vi "Generacion.vi"() -> ()   [LabVIEW 2016]
uses:
  <vilib>/sound2/lvsound2.llb/Sound Data Format.ctl
  <vilib>/sound2/lvsound2.llb/Sampling Mode.ctl
  <vilib>/measure/NI_MABase.lvlib
  <vilib>/Waveform/WDTOps.llb/WDT Append Waveforms DBL.vi
  <vilib>/sound2/lvsound2.llb/Sound File Write (DBL Single).vi
  <vilib>/sound2/lvsound2.llb/Sound File Write Open.vi
  <vilib>/sound2/lvsound2.llb/Sound Output Write (DBL Single).vi
panel:
  out "size(s)":i32
  in  "Normalizar":bool caption="Normalizar amplitud"
  in  "Tipo fichero":T1(ring)
  in  "Generar":bool
  in  "Reproducir":bool
  in  "Exit":bool
  in  "Salvar":bool
  in  "Ruido":bool
  in  "A_ruido":dbl=0.1 caption="Amplitud ruido"
  in  "Tipo_portadora":T2(ring) caption="Tipo portadora"
  in  "A_portadora":dbl=0.7 caption="Amplitud portadora" min=0.0 max=1.0
  in  "T_portadoras":dbl[](array[numeric])=[100.0, 150.0, 100.0, 150.0, 100.0, 150.0, 100.0] caption="Tiempo entre portadoras (ms)"
  out "Señal":waveform(dbl)(graph)
  in  "Duración":dbl=5.0 caption="Duración portadora (ms)"
  in  "Muestreo":dbl=48000.0 caption="Muestreo (muestras/s)"
  in  "F_portadora":dbl=1000.0 caption="Frecuencia portadora (Hz)" format="%#_13g"
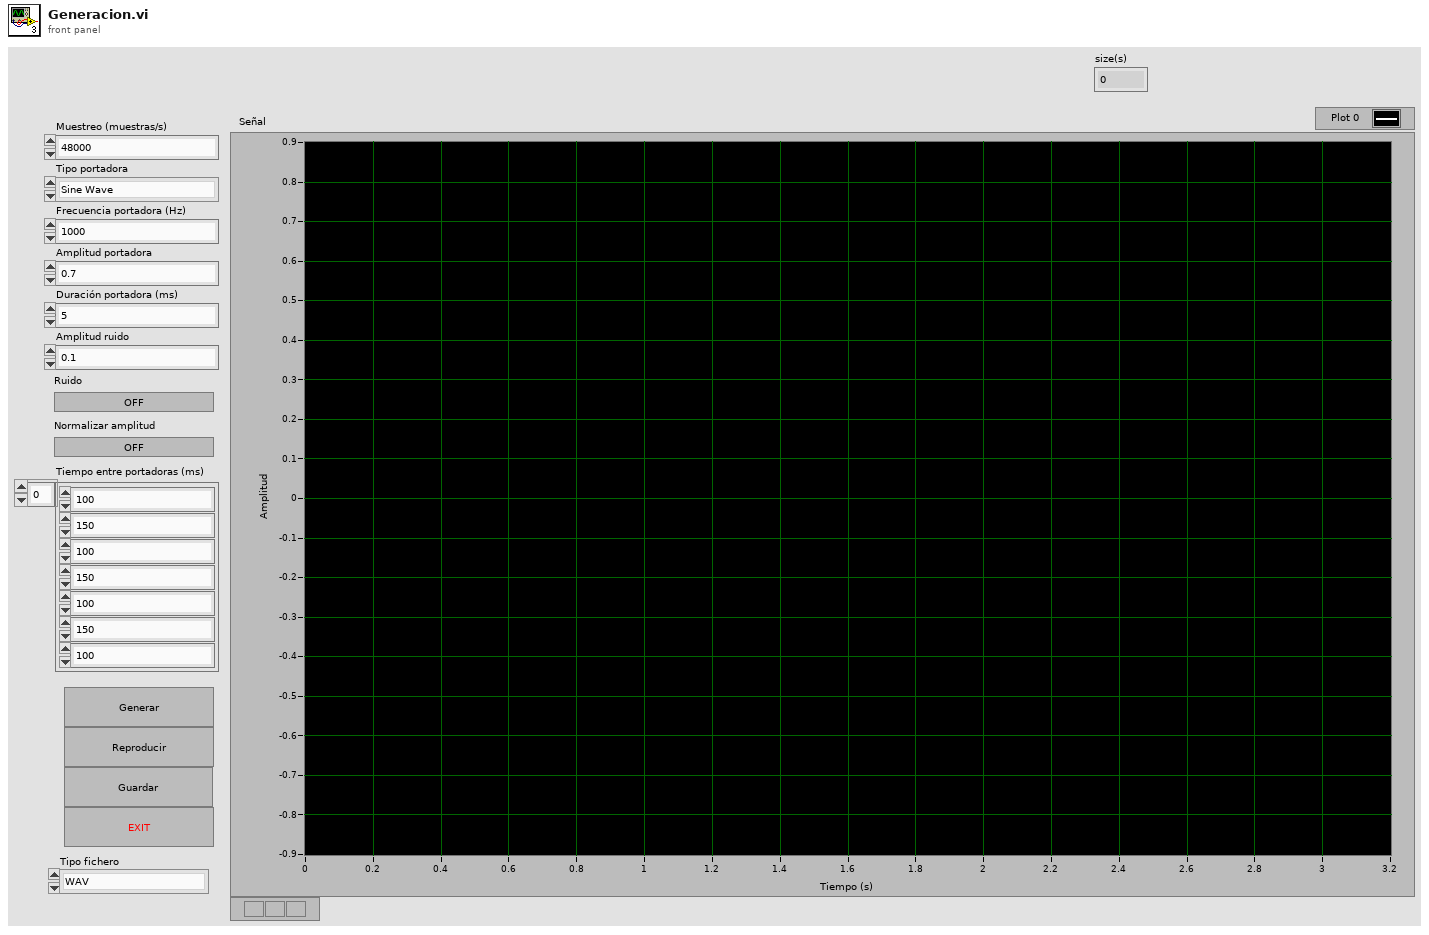
[diagram p1: front panel]
types:
  T1 = enum16{"WAV", "Bin 16 bits, little-endian", "Bin 16 bits, big-endian"}
  T2 = enum16{"Sine Wave", "Triangle Wave", "Square Wave", "Sawtooth Wave"}
  T3 = typedef "Sound Data Format.ctl" = cluster{"sample rate (S/s)":dbl, "number of channels":i32, "bits per sample":i32}
  T4 = enum16{"big-endian, network order", "native, host order", "little-endian"}
  T5 = enum16{"open", "replace", "create", "open or create", "replace or create", "replace or create with confirmation"}
  T6 = typedef "Sound File Refnum.ctl" = refnum<file>
  T7 = typedef "Sampling Mode.ctl" = i32
  T8 = typedef "Sound Output Task ID.ctl" = u32
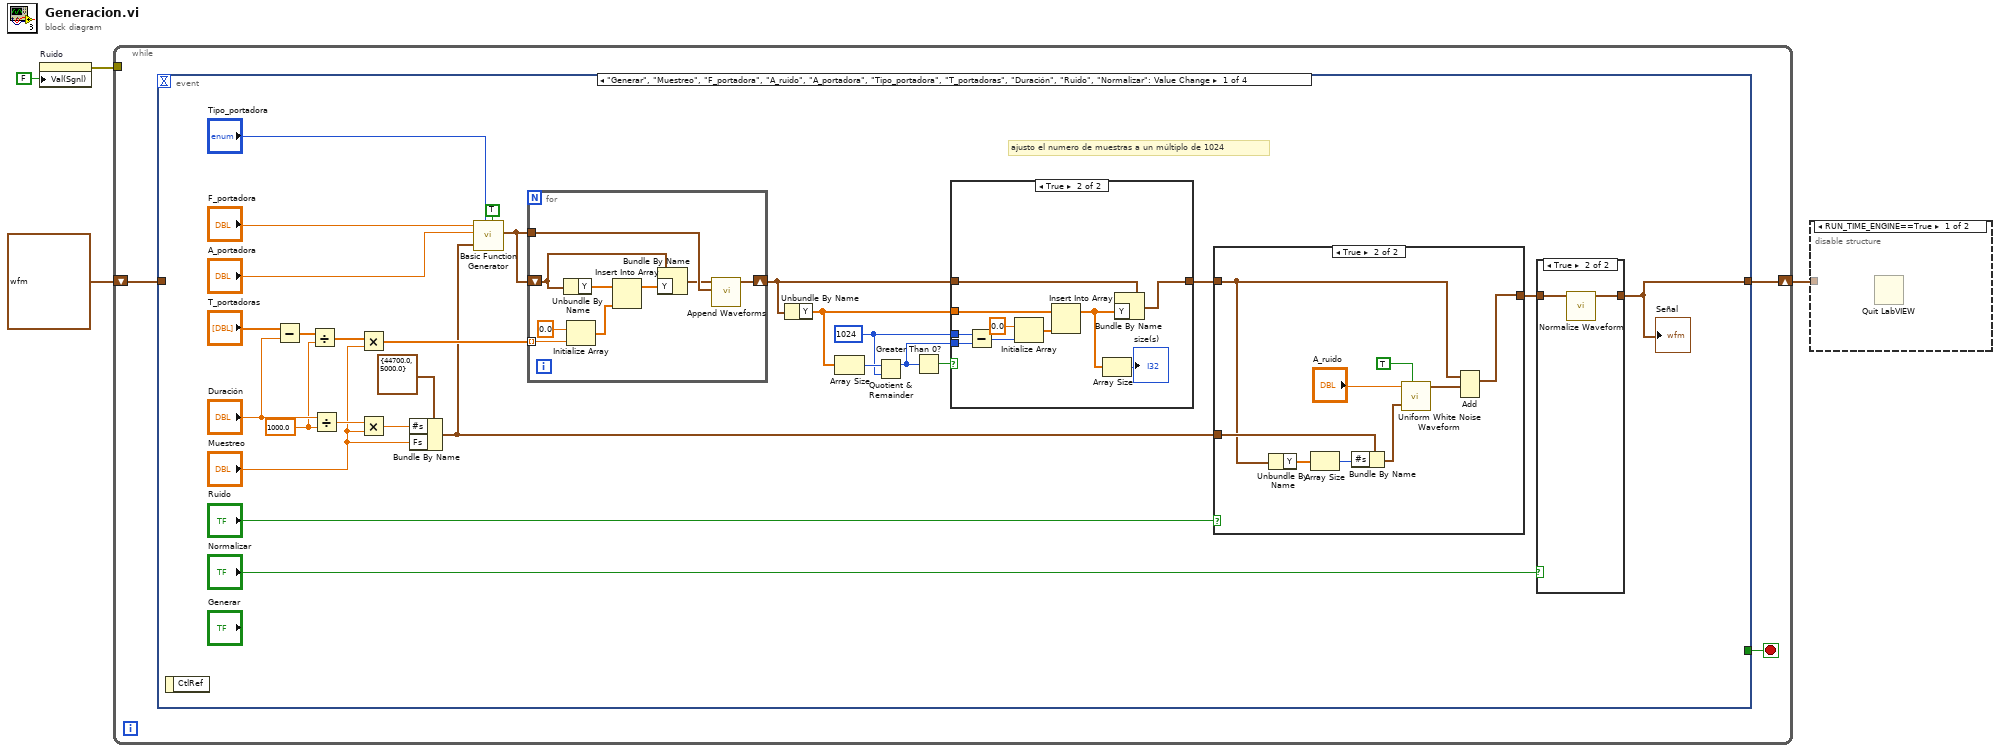
[diagram p0: block diagram]
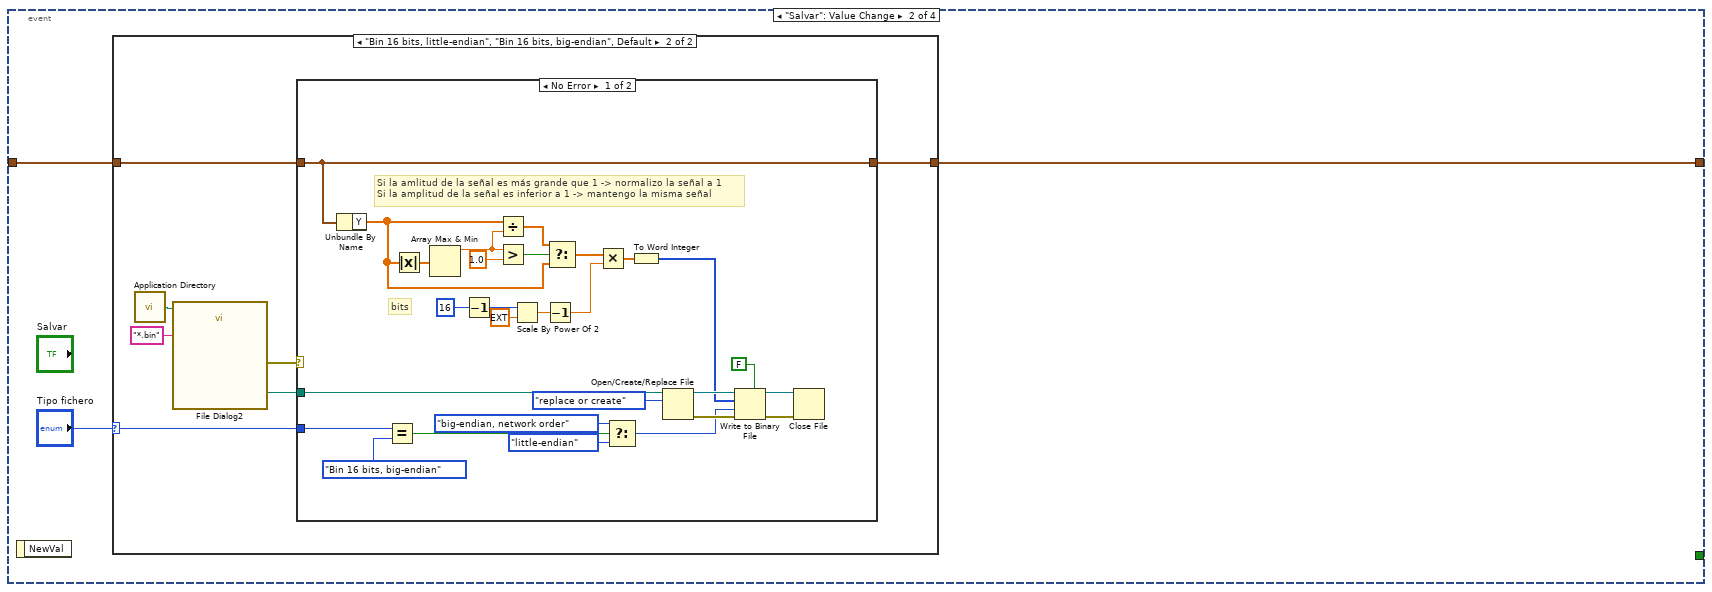
[diagram p6: hidden frame]
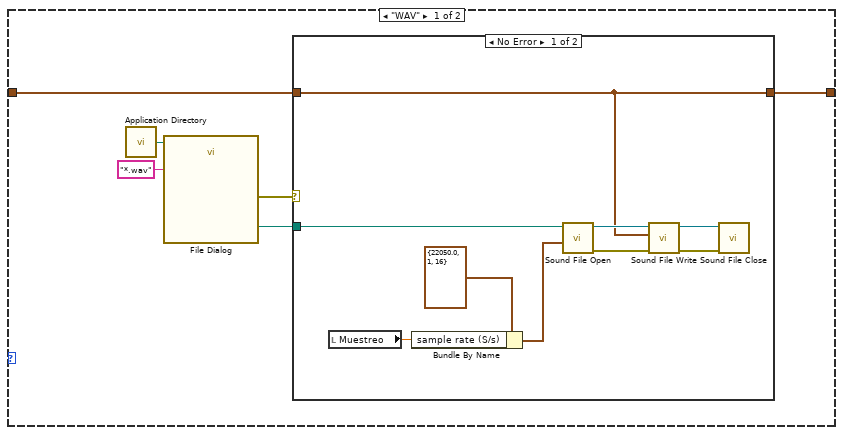
[diagram p7: hidden frame]
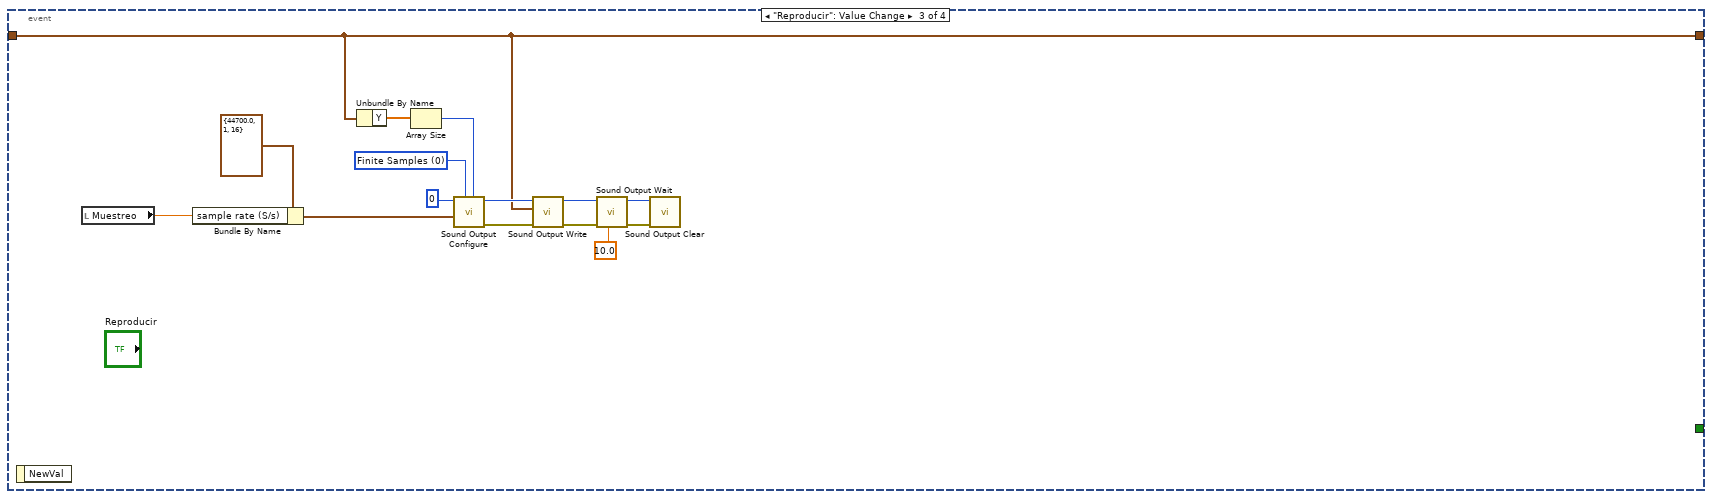
[diagram p10: hidden frame]
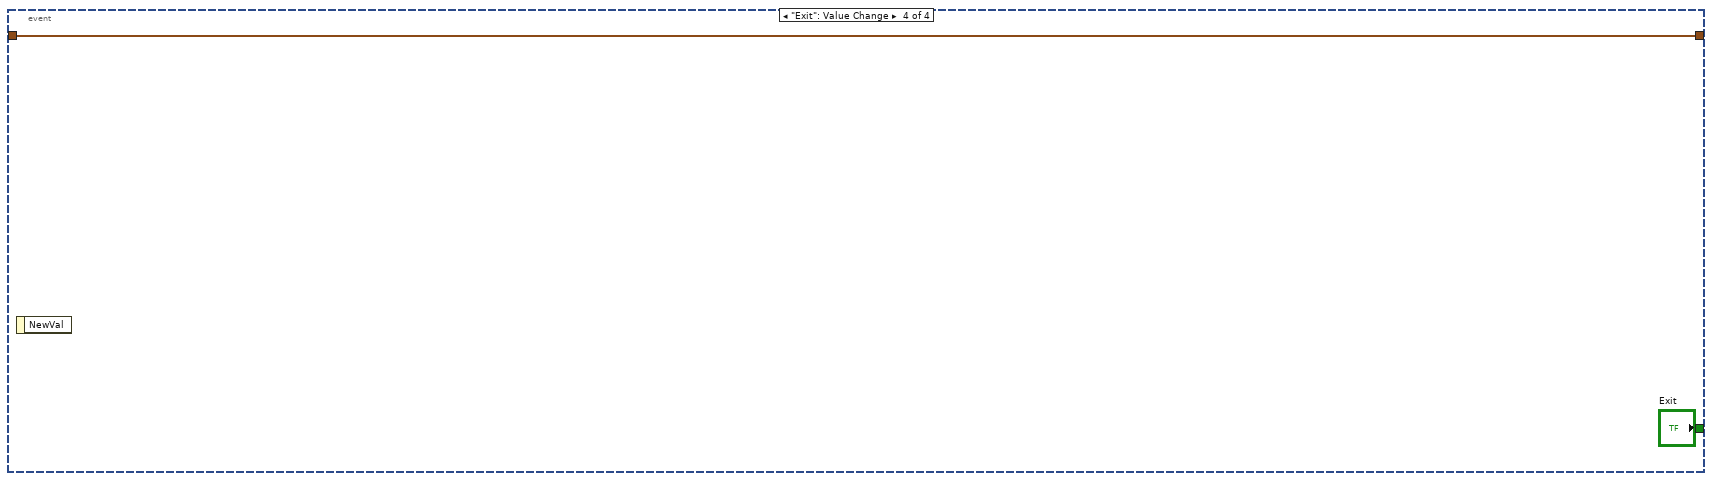
[diagram p11: hidden frame]
diagram:
  n1 = property on="Ruido" class="Bool (strict)"("Val(Sgnl)"=FALSE ("Value (Signaling)")) -> (error out=w3:errorcluster)  [unwired: 2 in, 1 out]
  n2 = while {
    shift-right: [w6] -> w1
    shift-left: waveform(dbl) {"t0"=timestamp(0 s since 1904-01-01), "dt"=1.0, "Y"=[]} ("signal out") -> [w5]
    tunnel: w3 -> [_]
    stop <- w7 stop-if-true
    n3 = event shown="[0] \"Generar\", \"Muestreo\", \"F_portadora\", \"A_ruido\", \"A_portadora\", \"Tipo_portadora\", \"T_portadoras\", \"Duración\", \"Ruido\", \"Normalizar\": Value Change" {
      selector: _ -> [_ _ _ _]
      dyn-events: _ -> [_ _ _ _]
      timeout: _ -> [_ _ _ _]
      tunnel: [_ _ _ "Exit"] -> w7
      tunnel: [w17 w68 w126 w138] -> w6
      tunnel: w5 -> [_ w69 w126 w138]
      event "Generar", "Muestreo", "F_portadora", "A_ruido", "A_portadora", "Tipo_portadora", "T_portadoras", "Duración", "Ruido", "Normalizar": Value Change {
        w8 = 1024 ("y")
        w16 = 1000.0 ("y")
        # "ajusto el numero de muestras a un múltiplo de 1024"
        n4 = event-data() -> ()  [unwired: 1 in, 1 out]
        n5 = Subtract(x="T_portadoras", y="Duración") -> (x-y=w28:dbl[])
        n6 = Divide(x=w28, y=w16) -> (x/y=w32:dbl[])
        n7 = Divide(x="Duración", y=w16) -> (x/y=w34:dbl)
        n8 = Multiply(x=w32, y="Muestreo") -> (x*y=w31:dbl[])
        n9 = Multiply(x=w34, y="Muestreo") -> (x*y=w33:dbl)
        n10 = Bundle By Name(cluster=cluster{"Fs":dbl, "#s":dbl} {"Fs"=44700.0, "#s"=5000.0} ("sampling info"), "#s"=w33, "Fs"="Muestreo") -> (w20:cluster{"Fs":dbl, "#s":dbl})
        n11 = call <vilib>:"Basic Function Generator.vi"("reset signal"=TRUE, "sampling info"=w20, "signal type"="Tipo_portadora", "amplitude"="A_portadora", "frequency"="F_portadora") -> ("signal out"=w26:waveform(dbl))  [unwired: 4 in, 2 out]
        n12 = for {
          shift-right: [w67] -> w12
          shift-left: w26 -> [w62]
          tunnel: w26 -> [w66]
          tunnel: w31 -> [w65] mode=indexing
          n13 = Unbundle By Name(w62) -> ("Y"=w59:dbl[])
          n14 = Initialize Array(0.0, w65) -> (w63:dbl[])
          n15 = Insert Into Array(array=w59, new element=w63) -> (w61:dbl[])  [unwired: 1 in]
          n16 = Bundle By Name(cluster=w62, "Y"=w61) -> (w60:waveform(dbl))
          n17 = call-poly <vilib>:"Append Waveforms.vi"("waveform B"=w66, "waveform A"=w60) -> ("waveform out"=w67:waveform(dbl))  [unwired: 8 in, 1 out]
        }
        n18 = Unbundle By Name(w12) -> ("Y"=w10:dbl[])
        n19 = Array Size(array=w10) -> (size(s)=w14:i32)
        n20 = Quotient & Remainder(x=w14, y=w8) -> (x-y*floor(x/y)=w11:i32)  [unwired: 1 out]
        n21 = Greater Than 0?(x=w11) -> (x > 0?=w13:bool)
        n22 = case shown="True" w13 {
          tunnel: w12 -> [w35 w42]
          tunnel: w11 -> [_ w38]
          tunnel: w10 -> [_ w45]
          tunnel: [w35 w41] -> w9
          tunnel: w8 -> [_ w37]
          frame False {
          }
          frame True {
            n23 = Subtract(x=w37, y=w38) -> (x-y=w36:i32)
            n24 = Initialize Array(0.0, w36) -> (w43:dbl[])
            n25 = Insert Into Array(array=w45, new element=w43) -> (w40:dbl[])  [unwired: 1 in]
            n26 = Array Size(array=w40) -> (size(s)=→"size(s)":i32)
            n27 = Bundle By Name(cluster=w42, "Y"=w40) -> (w41:waveform(dbl))
          }
        }
        n28 = case shown="True" "Ruido" {
          tunnel: w20 -> [_ w58]
          tunnel: [w49 w53] -> w18
          tunnel: w9 -> [w49 w50]
          frame False {
          }
          frame True {
            n29 = Unbundle By Name(w50) -> ("Y"=w56:dbl[])
            n30 = Array Size(array=w56) -> (size(s)=w55:i32)
            n31 = Bundle By Name(cluster=w58, "#s"=w55) -> (w57:cluster{"Fs":dbl, "#s":dbl})
            n32 = call <vilib>:"Uniform White Noise Waveform.vi"("sampling info"=w57, "reset signal"=TRUE, "amplitude"="A_ruido") -> ("signal out"=w54:waveform(dbl))  [unwired: 7 in, 1 out]
            n33 = Add(1:w54, 2:w50) -> (0:w53:waveform(dbl))  [unwired: 1 in, 1 out]
          }
        }
        n34 = case shown="True" "Normalizar" {
          tunnel: w18 -> [w46 w48]
          tunnel: [w46 w47] -> w17
          frame False {
          }
          frame True {
            n35 = call <vilib>:"Normalize Waveform.vi"("waveform in"=w48) -> ("normalized waveform"=w47:waveform(dbl))  [unwired: 7 in, 3 out]
          }
        }
        "Señal" <- w17
      }
      event "Salvar": Value Change {
        n36 = event-data() -> ()  [unwired: 1 in, 1 out]
        n37 = case shown="\"Bin 16 bits, little-endian\", \"Bin 16 bits, big-endian\", Default" "Tipo fichero" {
          selector: "Tipo fichero" -> [_ w90]
          tunnel: w69 -> [w72 w89]
          tunnel: [w71 w88] -> w68
          frame "WAV" {
            n38 = call <vilib>:"Application Directory.vi"() -> ("Application Directory"=w73:path)
            n39 = call "File Dialog"("start path"=w73, "pattern (all files)"="*.wav") -> ("selected path"=w76:path, "error out"=w74:errorcluster)  [unwired: 10 in, 2 out]
            n40 = case shown="No Error" w74 {
              tunnel: w76 -> [w79 _]
              tunnel: w72 -> [w77 w86]
              tunnel: [w77 w86] -> w71
              frame No Error {
                n41 = local read "Muestreo"() -> (w78:dbl)
                n42 = Bundle By Name(cluster=T3 {"sample rate (S/s)"=22050.0, "number of channels"=1, "bits per sample"=16} ("sound format"), "sample rate (S/s)"=w78) -> (w80:T3)
                n43 = call-poly <vilib>:"Sound File Open.vi"("sound format"=w80, "path"=w79) -> ("error out"=w83:errorcluster, "sound file refnum"=w85:T6)  [unwired: 8 in]
                n44 = call-poly <vilib>:"Sound File Write.vi"("error in (no error)"=w83, "data"=w77, "sound file refnum"=w85) -> ("error out"=w82:errorcluster, "sound file refnum out"=w84:T6)  [unwired: 7 in]
                n45 = call <vilib>:"Sound File Close.vi"("error in (no error)"=w82, "sound file refnum"=w84) -> ()  [unwired: 9 in, 1 out]
              }
              frame Error {
              }
            }
          }
          frame "Bin 16 bits, little-endian", "Bin 16 bits, big-endian", Default {
            n46 = call <vilib>:"Application Directory.vi"() -> ("Application Directory"=w87:path)
            n47 = call "File Dialog2"("start path"=w87, "pattern (all files)"="*.bin") -> ("selected path"=w92:path, "error out"=w91:errorcluster)  [unwired: 10 in, 2 out]
            n48 = case shown="No Error" w91 {
              tunnel: w92 -> [w113 _]
              tunnel: w90 -> [w100 _]
              tunnel: w89 -> [w94 w122]
              tunnel: [w94 w122] -> w88
              frame No Error {
                # "Si la amlitud de la señal es más grande que 1 -> normalizo la señal a 1\nSi la amplitud de la señal es inferior a 1 -> mantengo la misma señal"
                # "bits"
                n49 = Unbundle By Name(w94) -> ("Y"=w101:dbl[])
                n50 = Equal?(x=w100, y=T1."Bin 16 bits, big-endian") -> (x = y?=w98:bool)
                n51 = Absolute Value(x=w101) -> (abs(x)=w109:dbl[])
                n52 = Array Max & Min(array=w109) -> (max value=w108:dbl)  [unwired: 3 out]
                n53 = Decrement(x=i16 16 ("n")) -> (x-1=w103:i16)
                n54 = Divide(x=w101, y=w108) -> (x/y=w106:dbl[])
                n55 = Greater?(x=w108, y=1.0) -> (0:w107:bool)
                n56 = Scale By Power Of 2(n=w103, x=ext 1.0) -> (x*2^n=w115:ext)
                n57 = Decrement(x=w115) -> (x-1=w114:ext)
                n58 = Select(t=w106, s=w107, f=w101) -> (s? t:f=w105:dbl[])
                n59 = Multiply(x=w105, y=w114) -> (x*y=w112:ext[])
                n60 = Select(t=T4."big-endian, network order" ("byte order (0:big-endian, network order)"), s=w98, f=T4."little-endian" ("byte order (0:big-endian, network order)")) -> (s? t:f=w95:T4)
                n61 = To Word Integer(number=w112) -> (16bit integer=w102:i16[])
                n62 = Open/Create/Replace File(file path (use dialog)=w113, operation (0:open)=T5."replace or create") -> (refnum out=w121:refnum<file>, error out=w120:errorcluster)  [unwired: 4 in, 1 out]
                n63 = Write to Binary File(file (use dialog)=w121, data=w102, error in=w120, 5:FALSE ("prepend array or string size? (T)"), 9:w95) -> (refnum out=w119:refnum<file>, error out=w118:errorcluster)  [unwired: 1 in, 1 out]
                n64 = Close File(refnum=w119, error in=w118) -> ()  [unwired: 2 out]
              }
              frame Error {
              }
            }
          }
        }
      }
      event "Reproducir": Value Change {
        w128 = T7 0 items=["Finite Samples", "Continuous Samples"] ("sample mode")
        n65 = event-data() -> ()  [unwired: 1 in, 1 out]
        n66 = local read "Muestreo"() -> (w123:dbl)
        n67 = Bundle By Name(cluster=T3 {"sample rate (S/s)"=44700.0, "number of channels"=1, "bits per sample"=16} ("sound format"), "sample rate (S/s)"=w123) -> (w137:T3)
        n68 = Unbundle By Name(w126) -> ("Y"=w125:dbl[])
        n69 = Array Size(array=w125) -> (size(s)=w124:i32)
        n70 = call <vilib>:"Sound Output Configure.vi"("number of samples/ch"=w124, "sample mode"=w128, "sound format"=w137, "device ID"=u32 0) -> ("error out"=w131:errorcluster, "task ID"=w132:T8)  [unwired: 6 in]
        n71 = call-poly <vilib>:"Sound Output Write.vi"("error in (no error)"=w131, "data"=w126, "task ID"=w132) -> ("error out"=w134:errorcluster, "task ID out"=w133:T8)  [unwired: 7 in]
        n72 = call <vilib>:"Sound Output Wait.vi"("timeout (sec)"=10.0, "error in (no error)"=w134, "task ID"=w133) -> ("error out"=w136:errorcluster, "task ID out"=w135:T8)  [unwired: 7 in]
        n73 = call <vilib>:"Sound Output Clear.vi"("error in (no error)"=w136, "task ID"=w135) -> ()  [unwired: 9 in, 1 out]
      }
      event "Exit": Value Change {
        n74 = event-data() -> ()  [unwired: 1 in, 1 out]
      }
    }
  }
  n75 = disable-structure shown="RUN_TIME_ENGINE==True" {
    disable-tunnel: w1 -> [_ _]
    frame condition #0 {
      n76 = Quit LabVIEW() -> ()  [unwired: 1 in]
    }
    frame condition #1 (active) {
    }
  }
